vi "ThrustReadout.vi"(0 "Handle In":i32, 1 "k":dbl, 2 "LP1 Pin":u16, 3 "error in":errorcluster, 4 "LabJack Supply":dbl) -> (5 "Voltage Reading":dbl, 6 "Thrust Reading [Newton]":dbl, 7 "Displacement Reading [meter]":dbl, 8 "error out":errorcluster)   [LabVIEW 2021]
panel:
  # "inputs"
  # "outputs"
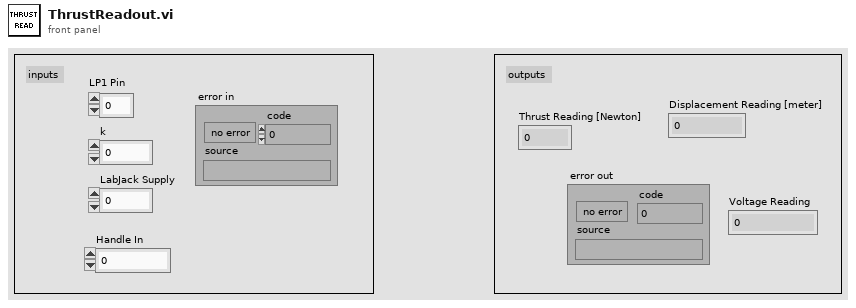
[diagram p1: front panel]
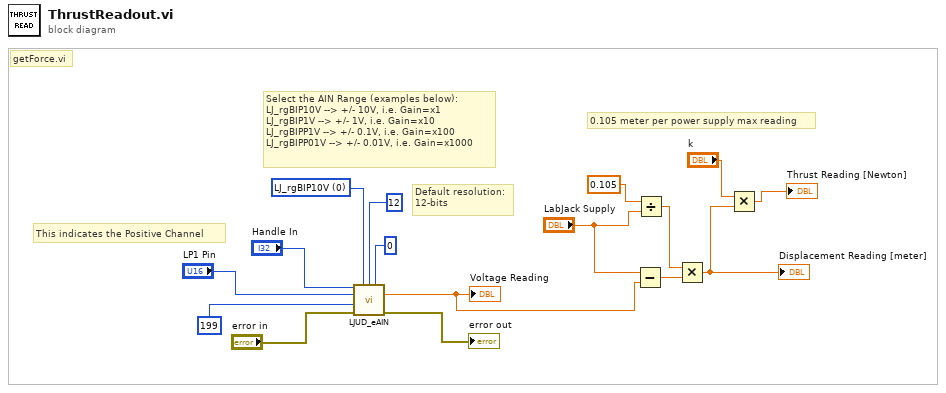
[diagram p0: block diagram]
diagram:
  w12 = u16 0 items=["LJ_rgBIP10V", "LJ_rgBIP1V", "LJ_rgBIPP1V", "LJ_rgBIPP01V"] ("AIN Range")
  # "0.105 meter per power supply max reading"
  # "getForce.vi"
  # "This indicates the Positive Channel"
  # "Default resolution:\n12-bits"
  # "Select the AIN Range (examples below):\nLJ_rgBIP10V --> +/- 10V, i.e. Gain=x1\nLJ_rgBIP1V --> +/- 1V, i.e. Gain=x10\nLJ_rgBIPP1V --> +/- 0.1V, i.e. Gain=x100\nLJ_rgBIPP01V --> +/- 0.01V, i.e. Gain=x1000"
  n1 = call <vilib>:"LJUD_eAIN.vi"("Handle In"="Handle In", "Range"=w12, "Resolution"=12, "Settling"=0, "ChannelP"="LP1 Pin", "ChannelN"=199, "error in"="error in") -> ("Voltage"=w2:dbl, "error out"=→"error out":errorcluster)  [unwired: 6 in, 1 out]
  "Voltage Reading" <- w2
  n2 = Subtract(x="LabJack Supply", y=w2) -> (x-y=w3:dbl)
  n3 = Divide(x=0.105, y="LabJack Supply") -> (x/y=w7:dbl)
  n4 = Multiply(x=w7, y=w3) -> (x*y=w5:dbl)
  "Displacement Reading [meter]" <- w5
  n5 = Multiply(x="k", y=w5) -> (x*y=→"Thrust Reading [Newton]":dbl)
